vi "Main.vi"() -> ()   [LabVIEW 2020]
panel:
  out "Application:Command Line Arguments":string[](array[string])
  in  "Start":bool
  out "current time":timestamp
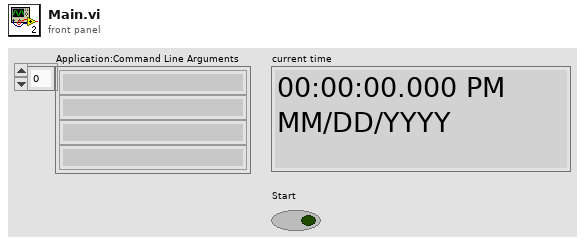
[diagram p1: front panel]
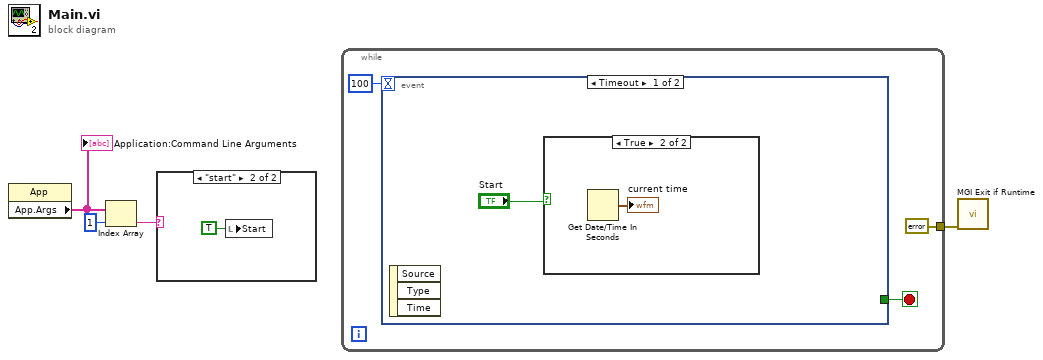
[diagram p0: block diagram]
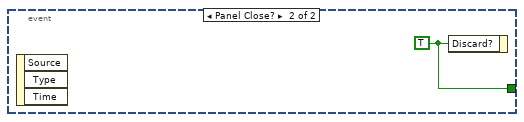
[diagram p4: hidden frame]
diagram:
  n1 = property class="App"() -> ("App.Args"=w3:string[])  [unwired: 2 in, 2 out]
  "Application:Command Line Arguments" <- w3
  n2 = Index Array(array=w3, index=1) -> (element=w1:string)
  n3 = case shown="\"start\"" w1 {
    frame "False", Default {
    }
    frame "start" {
      n4 = local write "Start"(TRUE ("Start")) -> ()
    }
  }
  n5 = while {
    tunnel: [errorcluster {"status"=FALSE, "code"=0, "source"=""} ("Error In (Dependency Only)")] -> w4
    stop <- w8 stop-if-true
    n6 = event shown="[0] Timeout" {
      selector: _ -> [_ _]
      dyn-events: _ -> [_ _]
      timeout: 100 -> [_ _]
      tunnel: [_ w11] -> w8
      event Timeout {
        n7 = event-data() -> ()  [unwired: 1 in, 3 out]
        n8 = case shown="True" "Start" {
          frame False {
          }
          frame True {
            n9 = Get Date/Time In Seconds() -> (seconds since 1Jan1904=→"current time":timestamp)
          }
        }
      }
      event Panel Close? {
        w11 = TRUE ("Discard?")
        n10 = event-data() -> ()  [unwired: 1 in, 3 out]
        n11 = event-data("Discard?"=w11) -> ()  [unwired: 1 in, 1 out]
      }
    }
  }
  n12 = call <userlib>:"MGI Exit if Runtime.vi"("Error In (Dependency Only)"=w4) -> ()  [unwired: 11 in]
